vi "MainANN.vi"() -> ()   [LabVIEW 2020]
uses:
  Global Variables/Trainning Done.vi
  Global Variables/Training_Status.vi
  <vilib>/FPGAPlugInAG/IC-3173/niLvFpga_Open_IC-3173.vi
  <vilib>/rvi/interface/common/dynamic/niFpgaDynamicAddResources.vi
  <vilib>/FPGAPlugInAG/Dynamic/niLvFpga_Run_Dynamic.vi
  <vilib>/Utility/error.llb/Error Cluster From Error Code.vi
  <vilib>/rvi/errors/niLvFpgaAdjustHostInterfaceError.vi
  <vilib>/FPGAPlugInAG/Dynamic/niLvFpga_Close_Dynamic.vi
  <vilib>/rvi/interface/nirviOpenFPGA/nirviOpenFPGA.xnode
  FPGA Bitfiles/recog_FPGATarget_FPGA-code_Tr10VxtkZqY.lvbitx
  FPGA-code.vi
  <vilib>/rvi/interface/nirviMethod/nirviMethod.xnode
  <vilib>/rvi/interface/nirviCloseFPGA/nirviCloseFPGA.xnode
  <vilib>/rvi/errors/niLvFpgaMergeErrorWithErrorCode.vi
  <vilib>/FPGAPlugInAG/Dynamic/niLvFpga_WriteFifo_Dynamic.vi
  <vilib>/FPGAPlugInAG/Dynamic/niLvFpga_ReadFifo_Dynamic.vi
panel:
  in  "Weights Mode":enum16{"", "Random Weights", "Prior Weights"}(ring)
  out "Updated Weights last trial":sgl[](array[numeric])
  out "Acc":dbl
  in  "?":sgl[](array[numeric])
  out "error out 3":errorcluster
  out "FPGA Close Error  2":errorcluster
  out "Intial Bias\n& Weights 2":dbl[](array[numeric])
  out "Classification":sgl[](array[numeric])
  out "Classification Input Layer":sgl[](array[numeric])
  out "trainingRecieved":bool
  in  "Mode":i32
  out "Read from FPGA Error 2":errorcluster
  out "Training Classification":sgl[](array[numeric])
  out "Elements Remaining FPGA queue 2":u32
  out "Empty Elements Remaining (control) 2":i16 format="%.5f"
  out "Reading Weights Error":errorcluster
  out "Queue empty":bool
  out "Received Weights and Biases":bool
  in  "Ready to Send":bool
  in  "Read Queue":bool=TRUE
  # "REMARK"
  # "To obtain the Weights the FPGA code has \nto be compiled first! Since the FIFO is flushed, \nimportant when running the logging VI."
  # "Training Data"
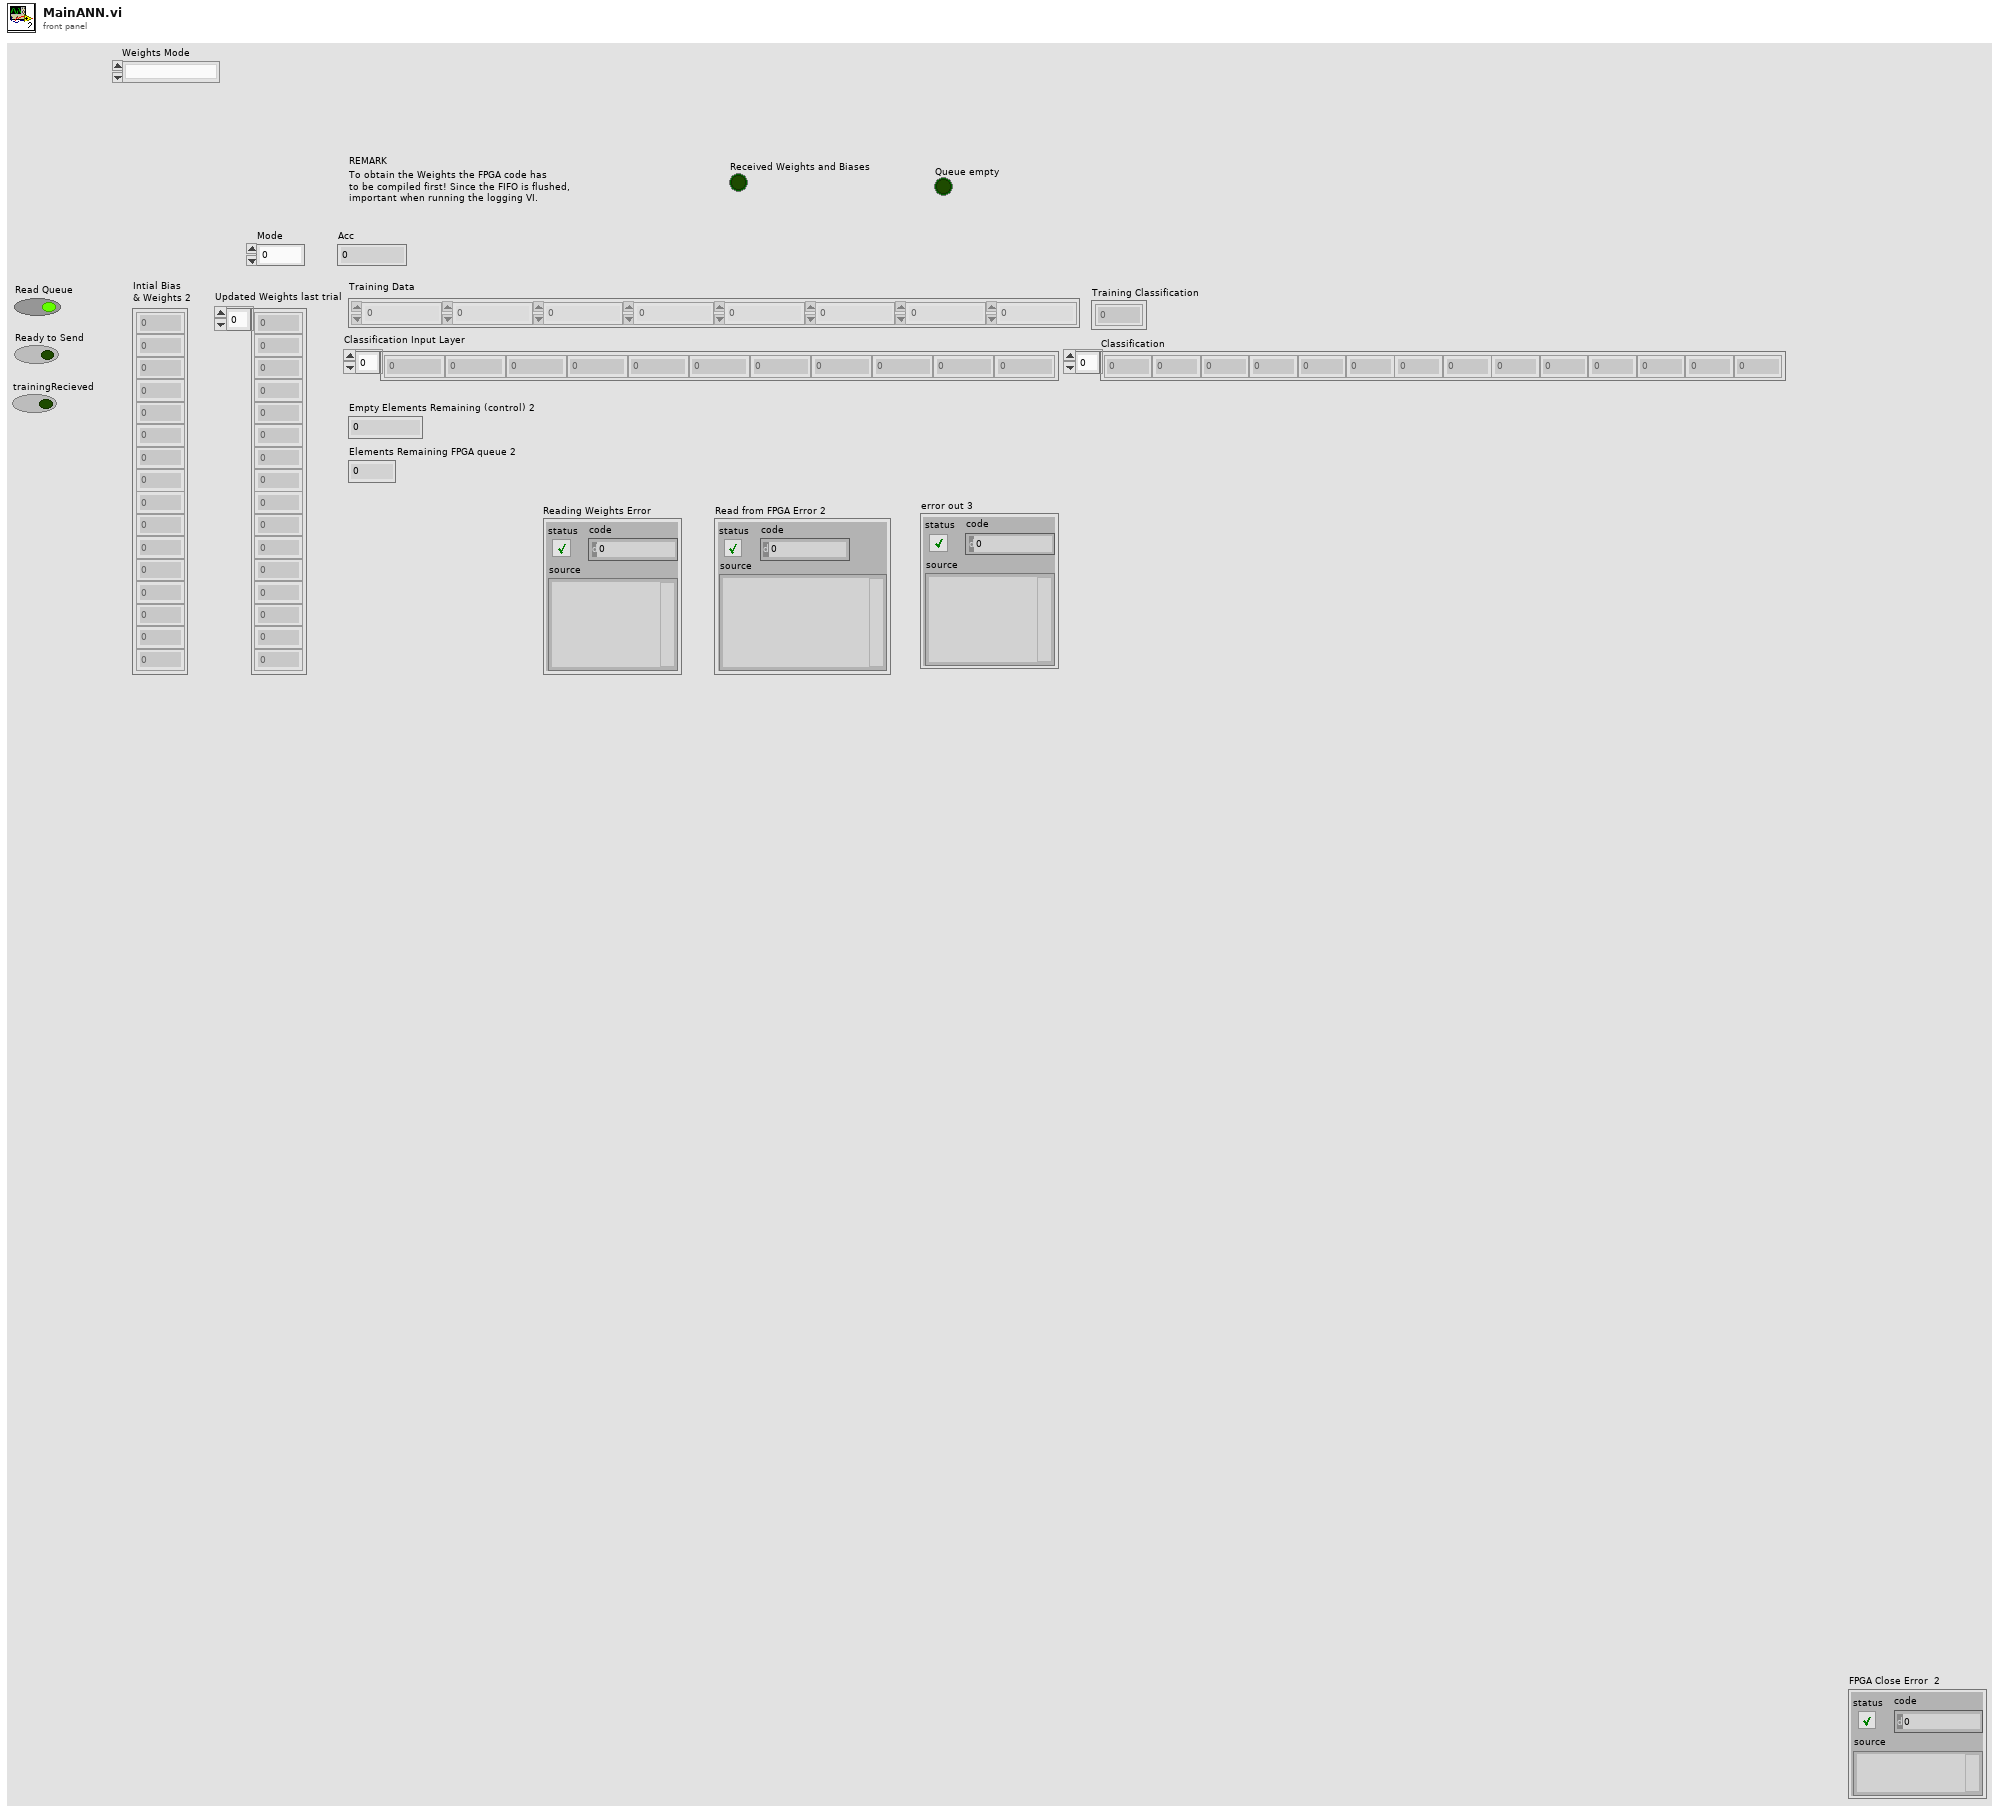
[diagram p1: front panel]
types:
  T1 = enum16{"open", "replace", "create", "open or create", "replace or create", "replace or create with confirmation"}
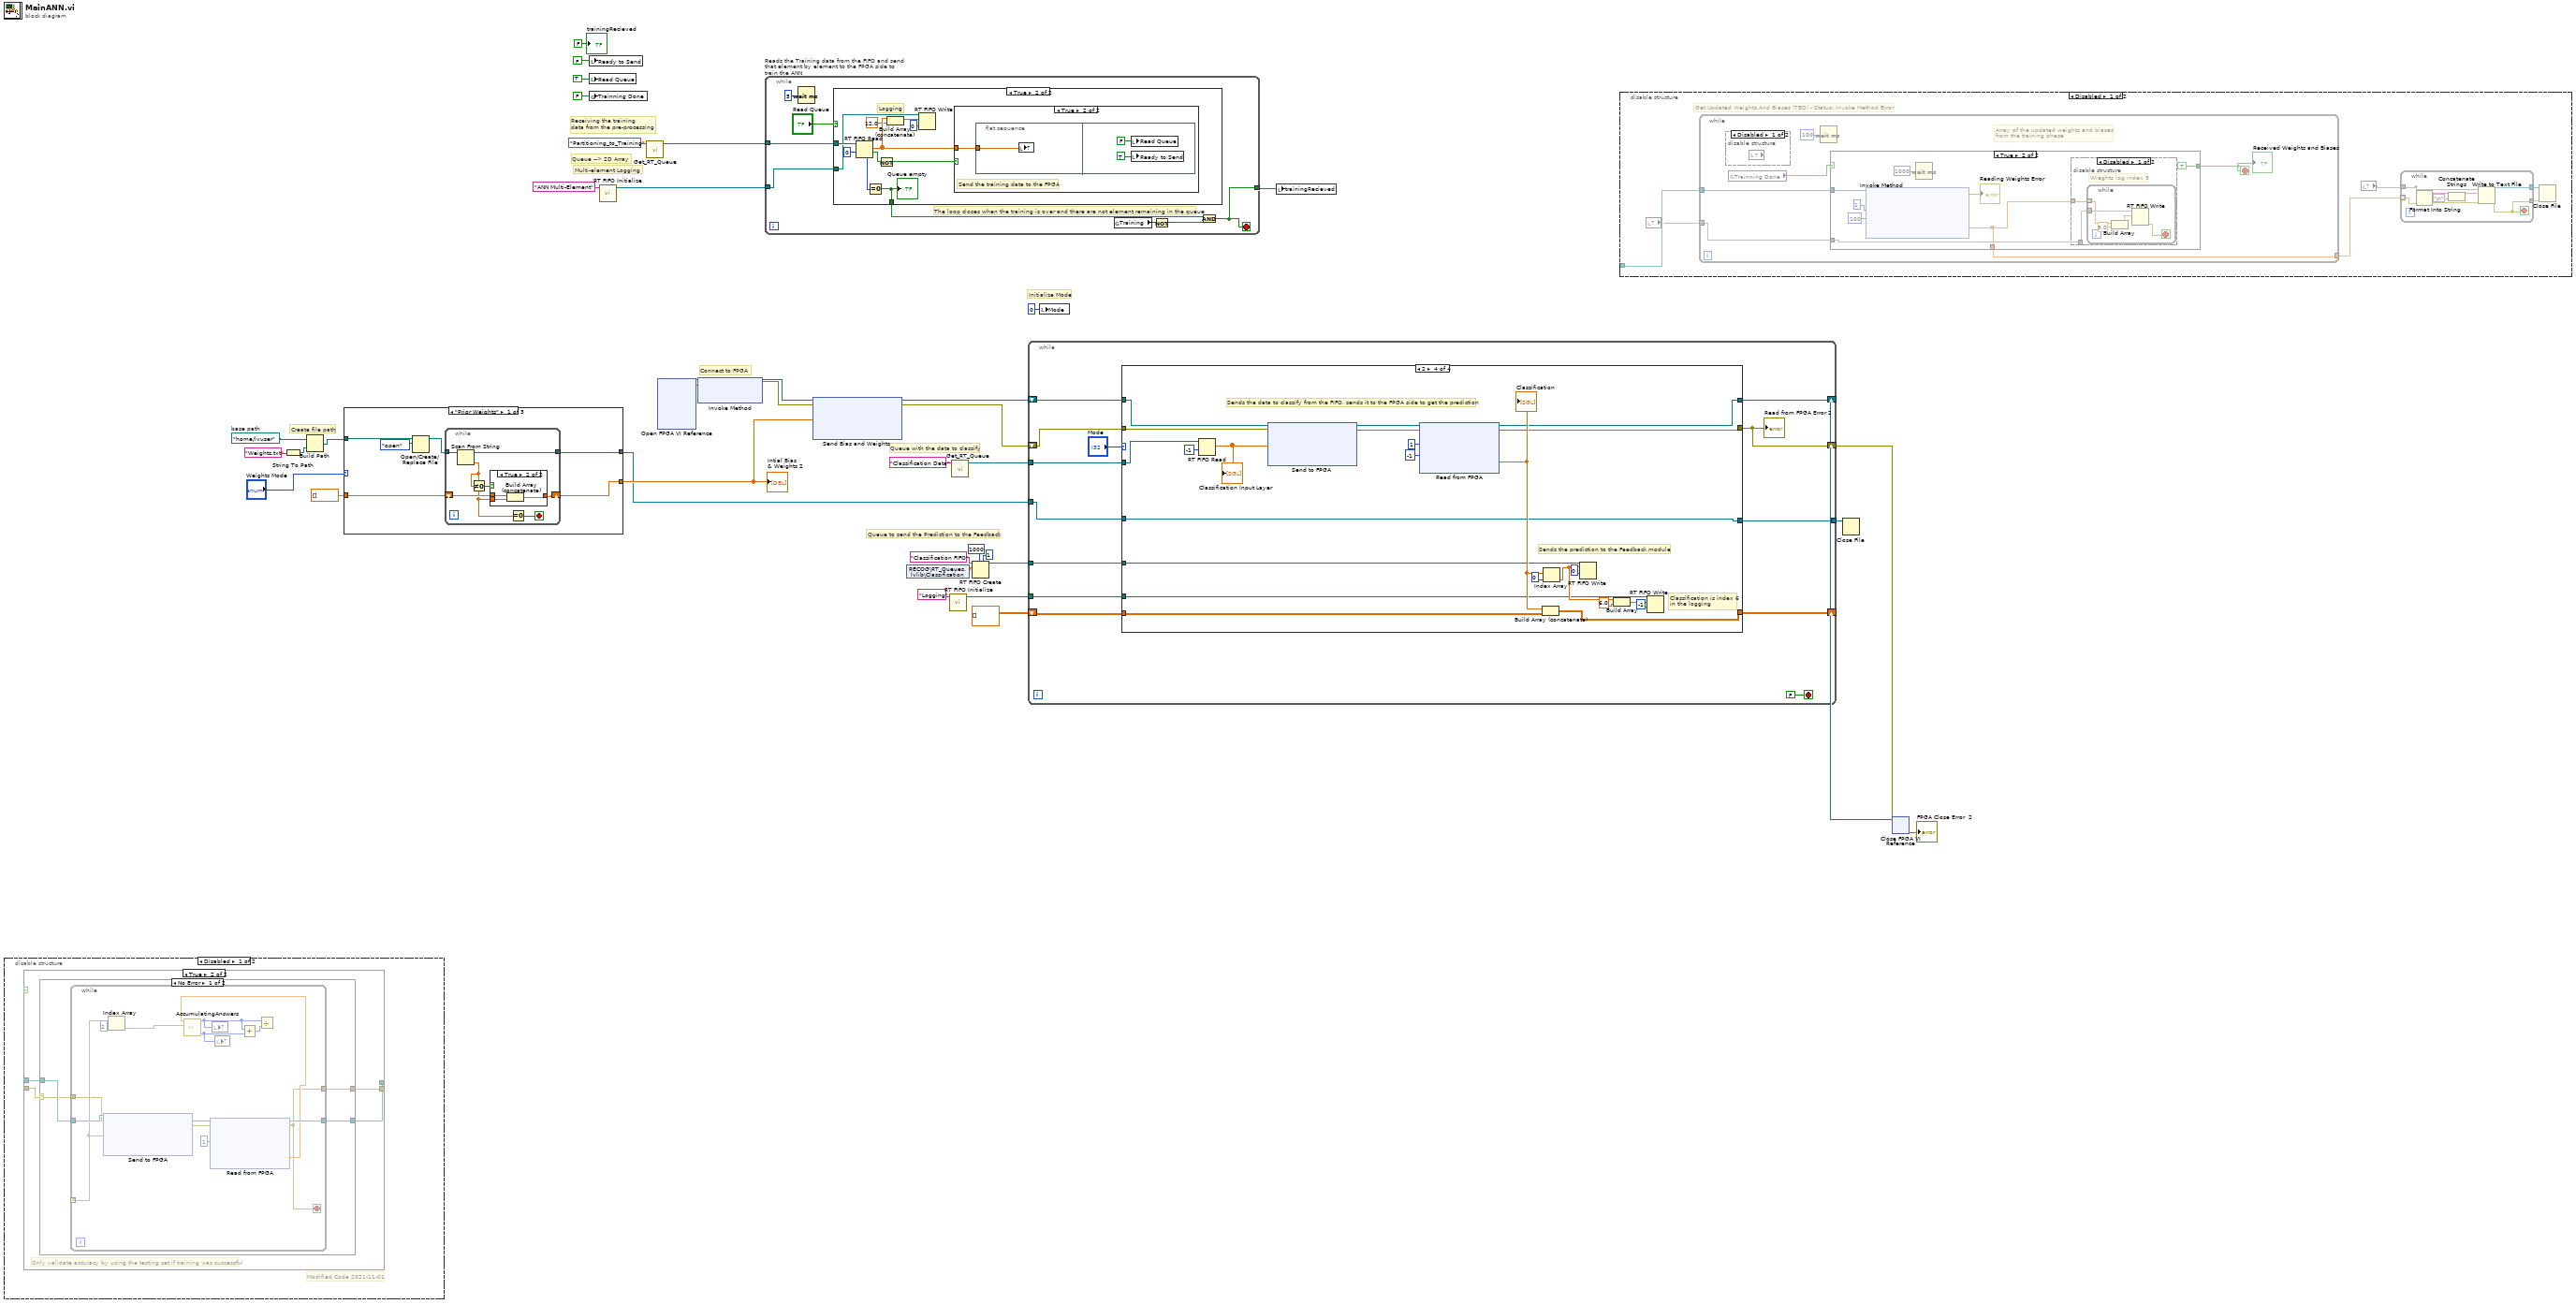
[diagram p0: block diagram]
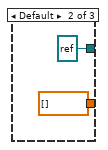
[diagram p3: hidden frame]
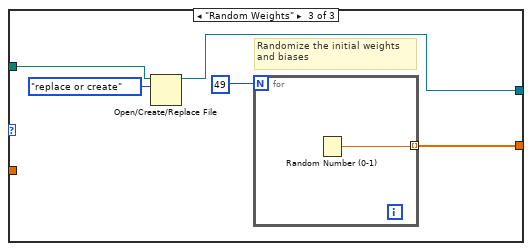
[diagram p4: hidden frame]
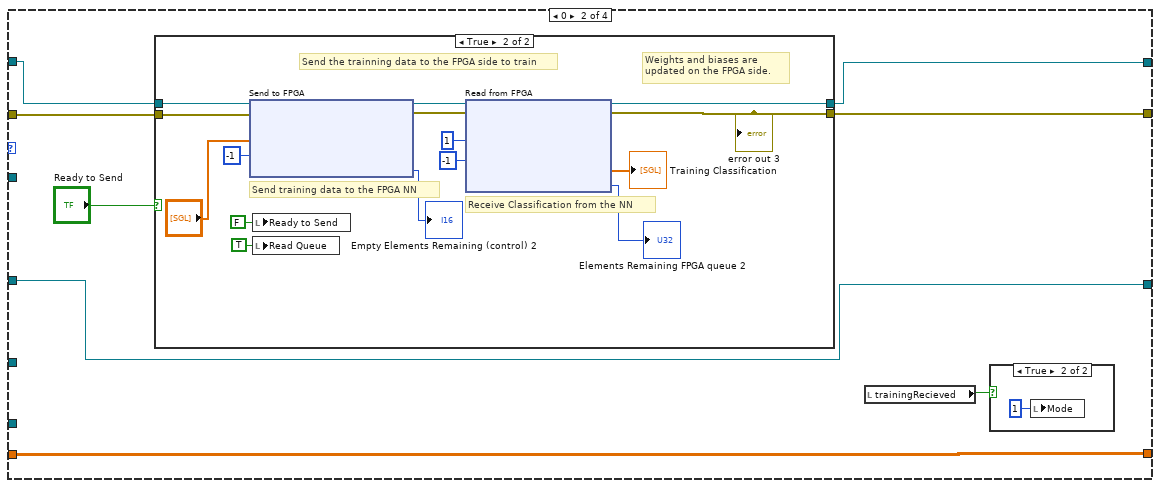
[diagram p6: hidden frame]
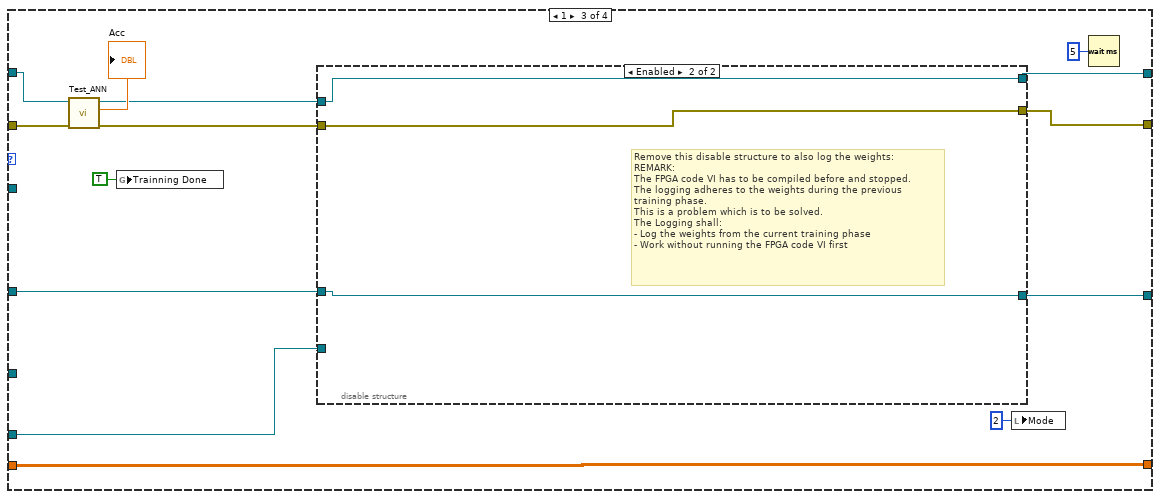
[diagram p9: hidden frame]
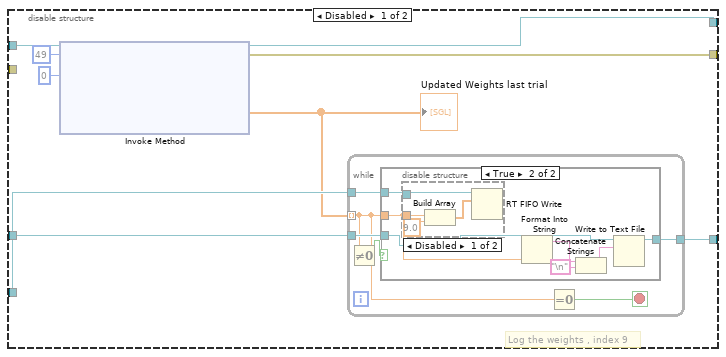
[diagram p10: hidden frame]
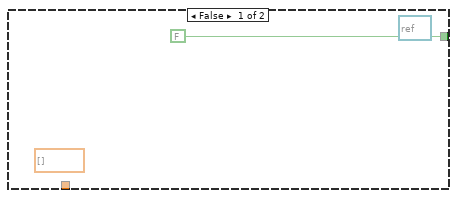
[diagram p14: hidden frame]
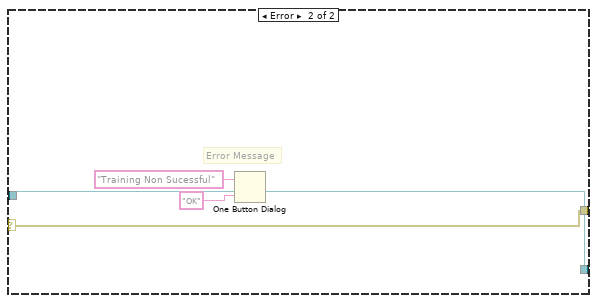
[diagram p18: hidden frame]
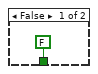
[diagram p20: hidden frame]
diagram:
  w8 = path "/home/lvuser"  # base path
  # "Create file path"
  # "Initialize Mode"
  # "Connect to FPGA"
  # "Queue with the data to classify"
  # "Queue to send the Prediction to the Feedback"
  # "Multi-element Logging"
  # "Receiving the training\ndata from the pre-processing"
  # "Queue --> 2D Array"
  n1 = disable-structure shown="Disabled" {
    frame Disabled {
      # "Modified Code 2021-11-01"
      n2 = case shown="True" {
        selector: _ -> [_ _]
        tunnel: [w40 w45] -> w39
        tunnel: _ -> [w40 w44]
        tunnel: _ -> [w41 w42]
        tunnel: [w41 w43] -> _
        frame False {
        }
        frame True {
          # "Only validate accuracy by using the testing set if training was successful"
          n3 = case shown="No Error" w42 {
            selector: w42 -> [w46 w70]
            tunnel: [w50 w71] -> w45
            tunnel: w44 -> [w49 w71]
            tunnel: [w47 w70] -> w43
            frame No Error {
              n4 = while {
                tunnel: [w54] -> w48 mode=indexing
                tunnel: [w51] -> w47
                tunnel: w46 -> [w52]
                tunnel: w49 -> [w57]
                tunnel: [w61] -> w50
                stop <- w51 stop-if-true
                n5 = xnode "Send to FPGA"("FPGA VI Reference In"=w57, "error in"=w52, "Data"=w54) -> ("FPGA VI Reference Out"=w58:refnum<k20>, "error out"=w59:errorcluster)  [unwired: 1 in, 1 out]
                n6 = Index Array(array=w54, index=2) -> (element=w53)
                n7 = xnode "Read from FPGA"("FPGA VI Reference In"=w58, "error in"=w59, "Number of Elements"=u32 1) -> ("FPGA VI Reference Out"=w61:refnum<k20>, "error out"=w51:errorcluster, "Data"=w60:sgl[])  [unwired: 1 in, 1 out]
                n8 = call "AccumulatingAnswers.vi"("Label"=w53, "Output"=w60) -> (0:"wrong"=w62:i32, 3:"right"=w63:i32, 8:"wrong"=w64:i32, 9:"right"=w65:i32)  [unwired: 6 in]
                n9 = local write item#-1(w63) -> ()
                n10 = local write item#-1(w62) -> ()
                n11 = Add(x=w63, y=w62) -> (x+y=w67:i32)
                n12 = Divide(x=w63, y=w67) -> (x/y=w66:dbl)
              }
            }
            frame Error {
              # "Error Message"
              n13 = One Button Dialog(message="Training Non Sucessful", button name ("OK")="OK") -> ()  [unwired: 1 out]
            }
          }
        }
      }
    }
    frame Enabled {
    }
  }
  n14 = String To Path(string="Weights.txt") -> (path=w7:path)
  n15 = Build Path(base path=w8, name or relative path=w7) -> (appended path=w5:path)
  n16 = case shown="\"Prior Weights\"" "Weights Mode" {
    tunnel: [w72 dbl[] [] w94] -> w18
    tunnel: w5 -> [w76 _ w92]
    tunnel: dbl[] [] -> [w74 _ _]
    tunnel: [w73 refnum<file> refnum ("refnum out") w91] -> w3
    frame "Prior Weights" {
      n17 = Open/Create/Replace File(file path (use dialog)=w76, operation (0:open)=T1."open") -> (refnum out=w75:refnum<file>)  [unwired: 4 in, 2 out]
      n18 = while {
        tunnel: w75 -> [w84]
        shift-right: [w81] -> w72
        shift-left: w74 -> [w82]
        tunnel: [w80] -> w73
        stop <- w83 stop-if-true
        n19 = Scan From String(w84) -> (w80:refnum<file>, output 1=w78:dbl)  [unwired: 3 in, 1 out]
        n20 = Not Equal To 0?(x=w78) -> (x != 0?=w79:bool)
        n21 = case shown="True" w79 {
          tunnel: w82 -> [w85 w88]
          tunnel: [w85 w87] -> w81
          tunnel: w78 -> [_ w86]
          frame False {
          }
          frame True {
            n22 = Build Array (concatenate)(w88, w86) -> (w87:dbl[])
          }
        }
        n23 = Equal To 0?(x=w78) -> (x = 0?=w83:bool)
      }
    }
    frame Default {
    }
    frame "Random Weights" {
      # "Randomize the initial weights \nand biases"
      n24 = Open/Create/Replace File(file path (use dialog)=w92, operation (0:open)=T1."replace or create") -> (refnum out=w91:refnum<file>)  [unwired: 4 in, 2 out]
      n25 = for {
        N: 49 -> [_]
        tunnel: [w96] -> w94 mode=indexing
        n26 = Random Number (0-1)() -> (number: 0 to 1=w96:dbl)
      }
    }
  }
  "Intial Bias\n& Weights 2" <- w18
  n27 = local write "Ready to Send"(FALSE ("Ready to Send")) -> ()
  n28 = local write "Read Queue"(TRUE ("Read Queue")) -> ()
  n29 = global write "Trainning Done.vi" "Trainning Done"(FALSE ("Trainning Done")) -> ()
  n30 = call "RT FIFO Initialize.vi"("name (unnamed)"="ANN Multi-Element") -> ("rt fifo"=w32:refnum<k33>)  [unwired: 9 in, 1 out]
  n31 = call "Get_RT_Queue.vi"("String"="Partitioning_to_Training") -> ("rt fifo single"=w37:refnum<k33>)  [unwired: 8 in, 2 out]
  n32 = xnode "Open FPGA VI Reference"() -> ("FPGA VI Reference Out"=w16:refnum<k20>, "error out"=w17:errorcluster)  [unwired: 2 in]
  n33 = xnode "Invoke Method"("FPGA VI Reference In"=w16, "error in"=w17) -> ("FPGA VI Reference Out"=w19:refnum<k20>, "error out"=w20:errorcluster)  [unwired: 1 in]
  n34 = while "Reads the Training data from the FIFO and send that element by element to the FPGA side to train the ANN" {
    tunnel: w37 -> [w102]
    tunnel: [w101] -> w30
    tunnel: w32 -> [w97]
    stop <- w101 stop-if-true
    # "The loop closes when the training is over and there are not element remaining in the queue"
    n35 = Wait (ms)(milliseconds to wait=u32 5) -> ()  [unwired: 1 out]
    n36 = case shown="True" "Read Queue" {
      tunnel: w102 -> [_ w114]
      tunnel: [FALSE w111] -> w100
      tunnel: w97 -> [_ w110]
      frame False {
      }
      frame True {
        # "Logging"
        n37 = RT FIFO Read(0:w114, 2:0 ("timeout in ms (0)")) -> (7:w113:u32, 9:w109:sgl[], 10:w116:bool)  [unwired: 2 in, 2 out]
        n38 = Equal To 0?(x=w113) -> (x = 0?=w111:bool)
        "Queue empty" <- w111
        n39 = Not(x=w116) -> (.not. x?=w115:bool)
        n40 = Build Array (concatenate)(w109, 12.0) -> (w107:dbl[])
        n41 = RT FIFO Write(0:w110, 1:w107, 2:0 ("timeout in ms (0)")) -> ()  [unwired: 2 in, 4 out]
        n42 = case shown="True" w115 {
          tunnel: w109 -> [_ w117]
          frame False {
          }
          frame True {
            # "Send the training data to the FPGA"
            n43 = flat-sequence {
              tunnel: w117 -> [w118]
              frame #0 {
                n44 = local write item#16(w118) -> ()
              }
              frame #1 {
                n45 = local write "Read Queue"(FALSE ("Read Queue")) -> ()
                n46 = local write "Ready to Send"(TRUE ("Send Array")) -> ()
              }
            }
          }
        }
      }
    }
    n47 = global read "Training_Status.vi" "Training"() -> (w99:bool)
    n48 = Not(x=w99) -> (.not. x?=w98:bool)
    n49 = And(x=w100, y=w98) -> (x .and. y?=w101:bool)
  }
  n50 = xnode "Send Bias and Weights"("FPGA VI Reference In"=w19, "error in"=w20, "Data"=w18) -> ("FPGA VI Reference Out"=w15:refnum<k20>, "error out"=w10:errorcluster)  [unwired: 1 in, 1 out]
  n51 = shared-variable "RECOG\\RT_Queues.lvlib\\Classification"() -> (w27:dbl)  [unwired: 1 in, 1 out]
  n52 = call "RT FIFO Initialize.vi"("name (unnamed)"="Logging") -> ("rt fifo"=w23:refnum<k33>)  [unwired: 9 in, 1 out]
  n53 = call "Get_RT_Queue.vi"("String"="Classification Data") -> ("rt fifo single"=w21:refnum<k33>)  [unwired: 8 in, 2 out]
  n54 = RT FIFO Create(0:"Classification FIFO" ("name (unnamed)"), 1:w27, 4:u32 1000 ("size (10)"), 6:u32 1 ("elements in array (1)")) -> (8:w22:refnum<k33>)  [unwired: 4 in, 2 out]
  n55 = while {
    tunnel: w23 -> [w132]
    tunnel: w22 -> [w131]
    tunnel: w21 -> [w130]
    shift-right: [w128] -> w11
    shift-left: w15 -> [w129]
    shift-right: [w126] -> _
    shift-left: sgl[][] [] -> [w125]
    shift-right: [w124] -> w12
    shift-left: w10 -> [w123]
    tunnel: w3 -> [w122]
    tunnel: [w121] -> w1
    stop <- FALSE stop-if-true
    n56 = case shown="2" "Mode" {
      tunnel: w123 -> [w136 w145 w177 w218]
      tunnel: w129 -> [w137 w144 w168 w219]
      tunnel: [w137 w143 w176 w210] -> w128
      tunnel: [w136 w142 w166 w211] -> w124
      tunnel: w132 -> [_ _ w171 w217]
      tunnel: w131 -> [_ _ _ w216]
      tunnel: w125 -> [w135 w141 w175 w215]
      tunnel: [w135 w141 w175 w214] -> w126
      tunnel: w130 -> [_ _ _ w209]
      tunnel: w122 -> [w134 w138 w170 w208]
      tunnel: [w134 w138 w169 w208] -> w121
      frame Default {
      }
      frame 0 {
        n57 = case shown="True" "Ready to Send" {
          tunnel: w145 -> [w147 w155]
          tunnel: w144 -> [w148 w154]
          tunnel: [w148 w153] -> w143
          tunnel: [w147 w150] -> w142
          frame False {
          }
          frame True {
            # "Send the trainning data to the FPGA side to train"
            # "Weights and biases are \nupdated on the FPGA side."
            # "Receive Classification from the NN"
            # "Send training data to the FPGA NN"
            n58 = xnode "Send to FPGA"("FPGA VI Reference In"=w154, "error in"=w155, "Data"="?", "Timeout (ms)"=-1) -> ("FPGA VI Reference Out"=w159:refnum<k20>, "error out"=w158:errorcluster, "Empty Elements Remaining"=→"Empty Elements Remaining (control) 2":u32)
            n59 = local write "Ready to Send"(FALSE ("Ready to Send")) -> ()
            n60 = local write "Read Queue"(TRUE ("Read Queue")) -> ()
            n61 = xnode "Read from FPGA"("FPGA VI Reference In"=w159, "error in"=w158, "Number of Elements"=u32 1, "Timeout (ms)"=-1) -> ("FPGA VI Reference Out"=w153:refnum<k20>, "error out"=w150:errorcluster, "Data"=→"Training Classification":sgl[], "Elements Remaining"=→"Elements Remaining FPGA queue 2":u32)
            "error out 3" <- w150
          }
        }
        n62 = local read "trainingRecieved"() -> (w139:bool)
        n63 = case shown="True" w139 {
          frame False {
          }
          frame True {
            n64 = local write "Mode"(1 ("Mode")) -> ()
          }
        }
      }
      frame 1 {
        n65 = call "Test_ANN.vi"("error in (no error)"=w177, "FPGA VI Reference In"=w168) -> ("error out"=w164:errorcluster, "Acc"=→"Acc":dbl, "FPGA VI Reference Out"=w165:refnum<k20>)  [unwired: 7 in]
        n66 = global write "Trainning Done.vi" "Trainning Done"(TRUE ("Trainning Done")) -> ()
        n67 = disable-structure shown="Enabled" {
          disable-tunnel: [w186 w207] -> w176
          disable-tunnel: w171 -> [w183 _]
          disable-tunnel: w170 -> [w181 w206]
          disable-tunnel: [w180 w206] -> w169
          disable-tunnel: [w179 w205] -> w166
          disable-tunnel: w165 -> [w178 w207]
          disable-tunnel: w164 -> [_ w205]
          frame Disabled {
            # "Log the weights , index 9"
            n68 = xnode "Invoke Method"("FPGA VI Reference In"=w178, "Number of Elements"=u32 49, "Timeout (ms)"=0) -> ("FPGA VI Reference Out"=w186:refnum<k20>, "error out"=w179:errorcluster, "Data"=w182:sgl[])  [unwired: 1 in, 1 out]
            "Updated Weights last trial" <- w182
            n69 = while {
              tunnel: w183 -> [w192]
              tunnel: w182 -> [w187] mode=indexing
              tunnel: w181 -> [w191]
              tunnel: [w190] -> w180
              stop <- w189 stop-if-true
              n70 = Not Equal To 0?(x=w187) -> (x != 0?=w188:bool)
              n71 = case shown="True" w188 {
                tunnel: w192 -> [_ w200]
                tunnel: w191 -> [w193 w197]
                tunnel: [w193 w196] -> w190
                tunnel: w187 -> [_ w194]
                frame False {
                }
                frame True {
                  n72 = disable-structure shown="Disabled" {
                    disable-tunnel: w200 -> [w204 _]
                    disable-tunnel: w194 -> [w201 _]
                    frame Disabled {
                      n73 = Build Array(w201, sgl 9.0 ("element")) -> (w202:sgl[])
                      n74 = RT FIFO Write(0:w204, 1:w202) -> ()  [unwired: 3 in, 4 out]
                    }
                    frame Enabled {
                    }
                  }
                  n75 = Format Into String(w194) -> (resulting string=w198:string)  [unwired: 3 in, 1 out]
                  n76 = Concatenate Strings(w198, "\n") -> (w195:string)
                  n77 = Write to Text File(file (use dialog)=w197, text=w195) -> (refnum out=w196:refnum<file>)  [unwired: 2 in, 2 out]
                }
              }
              n78 = Equal To 0?(x=w187) -> (x = 0?=w189:bool)
            }
          }
          frame Enabled {
            # "Remove this disable structure to also log the weights: \nREMARK: \nThe FPGA code VI has to be compiled before and stopped. \nThe logging adheres to the weights during the previous \ntraining phase. \nThis is a problem which is to be solved. \nThe Logging shall: \n- Log the weights from the current training phase \n- Work without running the FPGA code VI first"
          }
        }
        n79 = local write "Mode"(2 ("Mode")) -> ()
        n80 = Wait (ms)(milliseconds to wait=u32 5) -> ()  [unwired: 1 out]
      }
      frame 2 {
        # "Classification is index 6\nin the logging"
        # "Sends the prediction to the Feedback module"
        # "Sends the data to classify from the FIFO, sends it to the FPGA side to get the prediction"
        n81 = RT FIFO Read(0:w209, 2:-1 ("timeout in ms (0)")) -> (9:w212:sgl[])  [unwired: 2 in, 4 out]
        "Classification Input Layer" <- w212
        n82 = xnode "Send to FPGA"("FPGA VI Reference In"=w219, "error in"=w218, "Data"=w212) -> ("FPGA VI Reference Out"=w229:refnum<k20>, "error out"=w228:errorcluster)  [unwired: 1 in, 1 out]
        n83 = xnode "Read from FPGA"("FPGA VI Reference In"=w229, "error in"=w228, "Number of Elements"=u32 1, "Timeout (ms)"=-1 ("Number of Elements")) -> ("FPGA VI Reference Out"=w210:refnum<k20>, "error out"=w211:errorcluster, "Data"=w225:sgl[])  [unwired: 1 out]
        "Classification" <- w225
        n84 = Build Array (concatenate)(w225, w215) -> (w214:sgl[][])
        n85 = Index Array(array=w225, index=0) -> (element=w224:sgl)
        n86 = RT FIFO Write(0:w216, 1:w224, 2:0 ("timeout in ms (0)")) -> ()  [unwired: 2 in, 4 out]
        n87 = Build Array(w224, sgl 6.0 ("element")) -> (w222:sgl[])
        n88 = RT FIFO Write(0:w217, 1:w222, 2:-1 ("timeout in ms (0)")) -> ()  [unwired: 2 in, 4 out]
      }
    }
    "Read from FPGA Error 2" <- w124
  }
  n89 = local write "Mode"(0 ("Mode")) -> ()
  n90 = local write "trainingRecieved"(w30) -> ()
  n91 = disable-structure shown="Disabled" {
    disable-tunnel: _ -> [w236 _]
    frame Disabled {
      # "Get Updated Weights And Biases (TBD) - Status: Invoke Method Error"
      n92 = local read item#-1() -> (w235)
      n93 = while {
        tunnel: w236 -> [w249]
        tunnel: w235 -> [w247]
        tunnel: [w245] -> w231
        stop <- w248 stop-if-true
        # "Array of the updated weights and biases \nfrom the training phase"
        n94 = disable-structure shown="Disabled" {
          frame Disabled {
            n95 = local read item#-1() -> ()  [unwired: 1 out]
          }
          frame Enabled {
          }
        }
        n96 = global read "Trainning Done.vi" "Trainning Done"() -> (w246:bool)
        n97 = Wait (ms)(milliseconds to wait=u32 100) -> ()  [unwired: 1 out]
        n98 = case shown="True" w246 {
          tunnel: w249 -> [_ w259]
          tunnel: [FALSE TRUE] -> w248
          tunnel: w247 -> [_ w255]
          tunnel: [_ w252] -> w245
          frame False {
            (unwired) sgl[] [] ("Data")
            (unwired) refnum<k20> refnum ("FPGA VI Reference Out")
          }
          frame True {
            n99 = xnode "Invoke Method"("FPGA VI Reference In"=w259, "Number of Elements"=u32 1, "Timeout (ms)"=100) -> ("error out"=→"Reading Weights Error":errorcluster, "Data"=w252:sgl[])  [unwired: 1 in, 2 out]
            n100 = Wait (ms)(milliseconds to wait=u32 1000) -> ()  [unwired: 1 out]
            n101 = disable-structure shown="Disabled" {
              disable-tunnel: w255 -> [w261 _]
              disable-tunnel: w252 -> [w260 _]
              frame Disabled {
                # "Wieghts log index 9"
                n102 = while {
                  tunnel: w261 -> [w266]
                  tunnel: w260 -> [w265] mode=indexing
                  stop <- w262 stop-if-true
                  n103 = Build Array(w265, sgl 9.0 ("element")) -> (w263:sgl[])
                  n104 = RT FIFO Write(0:w266, 1:w263) -> (11:w262:errorcluster)  [unwired: 3 in, 3 out]
                }
              }
              frame Enabled {
              }
            }
          }
        }
        "Received Weights and Biases" <- w248
      }
      n105 = local read item#-1() -> (w232)
      n106 = while {
        tunnel: [w244] -> _
        tunnel: w232 -> [w244]
        tunnel: w231 -> [w243] mode=indexing
        tunnel: [w239] -> w233
        tunnel: [w237] -> w234
        stop <- w237 stop-if-true
        n107 = Format Into String(w243) -> (resulting string=w242:string, error out=w238:errorcluster)  [unwired: 3 in]
        n108 = Concatenate Strings(w242, "\n") -> (w241:string)
        n109 = Write to Text File(file (use dialog)=w244, text=w241, error in=w238) -> (refnum out=w239:refnum<file>, error out=w237:errorcluster)  [unwired: 1 in, 1 out]
      }
      n110 = Close File(refnum=w233, error in=w234) -> ()  [unwired: 2 out]
    }
    frame Enabled {
    }
  }
  n111 = Close File(refnum=w1) -> ()  [unwired: 1 in, 2 out]
  n112 = xnode "Close FPGA VI Reference"("FPGA VI Reference In"=w11, "error in"=w12) -> ("error out"=→"FPGA Close Error  2":errorcluster)
  "trainingRecieved" <- FALSE ("trainingRecieved")
